vi "Write Discard.vi"(6 "Discard?":refnum<notifier>, 11 "Populate Menu Msg in":refnum<class "Populate Menu Msg.lvclass">) -> (3 "Populate Menu Msg out":refnum<class "Populate Menu Msg.lvclass">)   [LabVIEW 2017, in "Populate Menu Msg.lvclass"]
uses:
  <vilib>/gpm_packages/@cs/Test-executive-builder/Source/Test Executive Builder View/Test Executive Builder View Messages/Populate Menu Msg/Populate Menu Msg.lvclass
  <vilib>/gpm_packages/@cs/Test-executive-builder/Source/Test Executive Builder View/Test Executive Builder View Messages/Populate Menu Msg/Populate Menu Msg.lvclass/Populate Menu Msg.ctl
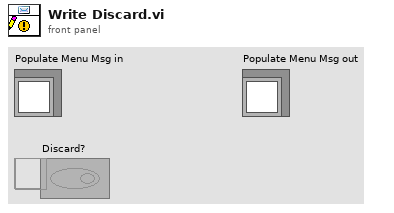
[diagram p1: front panel]
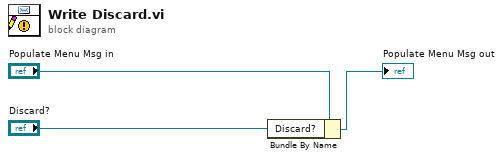
[diagram p0: block diagram]
diagram:
  n1 = Bundle By Name(cluster="Populate Menu Msg in", "Discard?"="Discard?") -> (→"Populate Menu Msg out":refnum<class "Populate Menu Msg.lvclass">)
